vi "Position Side Pane Tab.vi"(8 "error in (no error)":errorcluster, 10 "Flight Data (button Above)":refnum<vi>, 11 "Side Tab Ref":refnum<vi>) -> (0 "error out":errorcluster)   [LabVIEW 2014]
uses:
  Buttons/Standard button.ctl
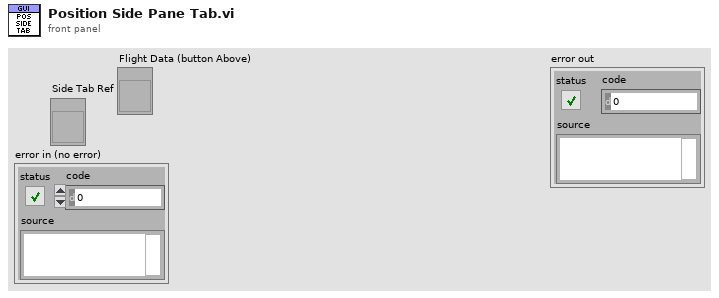
[diagram p1: front panel]
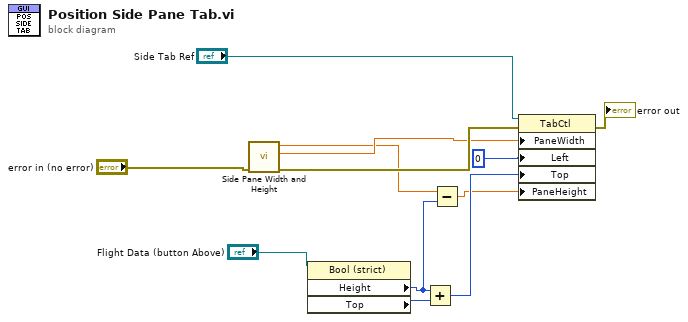
[diagram p0: block diagram]
diagram:
  n1 = call "Side Pane Width and Height.vi"("error in (no error)"="error in (no error)") -> ("error out"=w8:errorcluster, "Width"=w7:dbl, "Height"=w3:dbl)  [unwired: 8 in]
  n2 = property class="Bool (strict)"(reference="Flight Data (button Above)") -> ("Height"=w2:u32, "Top"=w5:i32)  [unwired: 1 in, 2 out]
  n3 = Add(x=w2, y=w5) -> (x+y=w4:u32)
  n4 = Subtract(x=w3, y=w2) -> (x-y=w1:dbl)
  n5 = property class="TabCtl"(reference="Side Tab Ref", error in=w8, "PaneWidth"=w7, "Left"=0 ("Position:Left"), "Top"=w4, "PaneHeight"=w1) -> (error out=→"error out":errorcluster)  [unwired: 1 out]
